vi "Labview-SortAFile .vi"() -> ()   [LabVIEW 2018]
panel:
  out "fichier trié":string[](array[string])
  out "spreadsheet string":string
  out "fichier":string[](array[string])
  out "text fichier liste.txt":string
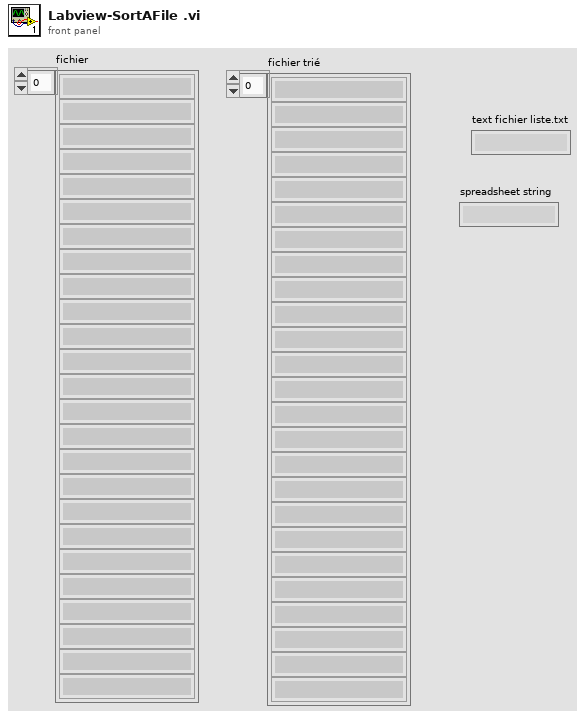
[diagram p1: front panel]
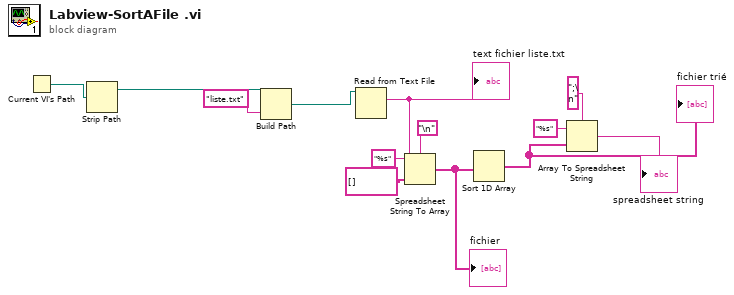
[diagram p0: block diagram]
diagram:
  n1 = Current VI's Path() -> (path=w13:path)
  n2 = Strip Path(path=w13) -> (stripped path=w12:path)  [unwired: 1 out]
  n3 = Build Path(base path=w12, name or relative path="liste.txt") -> (appended path=w10:path)
  n4 = Read from Text File(file (use dialog)=w10) -> (text=w7:string)  [unwired: 3 in, 3 out]
  "text fichier liste.txt" <- w7
  n5 = Spreadsheet String To Array(delimiter (Tab)="\n", format string="%s", spreadsheet string=w7, array type (2D Dbl)=string[] []) -> (array=w1:string[])
  "fichier" <- w1
  n6 = Sort 1D Array(array=w1) -> (sorted array=w2:string[])
  "fichier trié" <- w2
  n7 = Array To Spreadsheet String(delimiter (Tab)=";\n", array=w2, 3:"%s" ("format string")) -> (spreadsheet string=→"spreadsheet string":string)
